vi "OpenCVCam_Stop.vi"(8 "ErrorIn":errorcluster, 10 "CmdData":variant, 11 "OpenCVCamIn":refnum<class>) -> (0 "ErrorOut":errorcluster, 2 "ReplyData":variant, 3 "OpenCVCamOut":refnum<class>, 4 "Exit":bool)   [LabVIEW 2021, in "OpenCVCam.lvclass"]
uses:
  OpenCVCam.lvclass
  OpenCVCam.lvclass/OpenCVCam.ctl
  State.ctl
  C:/Localdata/Projects/TriekselSoft/TriekselsoftApplicationFramework/Source/.Externals/Library_YAF/YAFTAF/YAFTAF.lvclass
  C:/Localdata/Projects/TriekselSoft/TriekselsoftApplicationFramework/Source/.Externals/Library_YAF/YActor/YActor.lvclass
  C:/Localdata/Projects/TriekselSoft/TriekselsoftApplicationFramework/Source/.Externals/Interface_UserInterface_IFrontPanel/IFrontPanel/IFrontPanel.lvclass
  C:/Localdata/Projects/TriekselSoft/TriekselsoftApplicationFramework/Source/IInterface/IInterface.lvclass
  C:/Localdata/Projects/TriekselSoft/TriekselsoftApplicationFramework/Source/.Externals/Interface_Object_ICreateDestroy/ICreateDestroy/ICreateDestroy.lvclass
  C:/Localdata/Projects/TriekselSoft/TriekselsoftApplicationFramework/Source/.Externals/Interface_Object_IPersistentData/IPersistentData/IPersistentData.lvclass
  C:/Localdata/Projects/TriekselSoft/TriekselsoftApplicationFramework/Source/.Externals/Interface_TAF_ITAFObject/ITAFObject/ITAFObject.lvclass
  C:/Localdata/Projects/TriekselSoft/TriekselsoftApplicationFramework/Source/YAFTAFObjects/OpenCVCam/OpenCVCam.lvclass
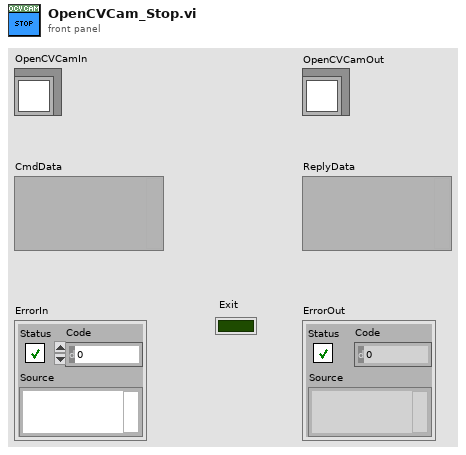
[diagram p1: front panel]
types:
  T1 = typedef "OpenCVCam.lvclass/State.ctl" = enum16{"Idle", "Initialized", "Acquiring"}
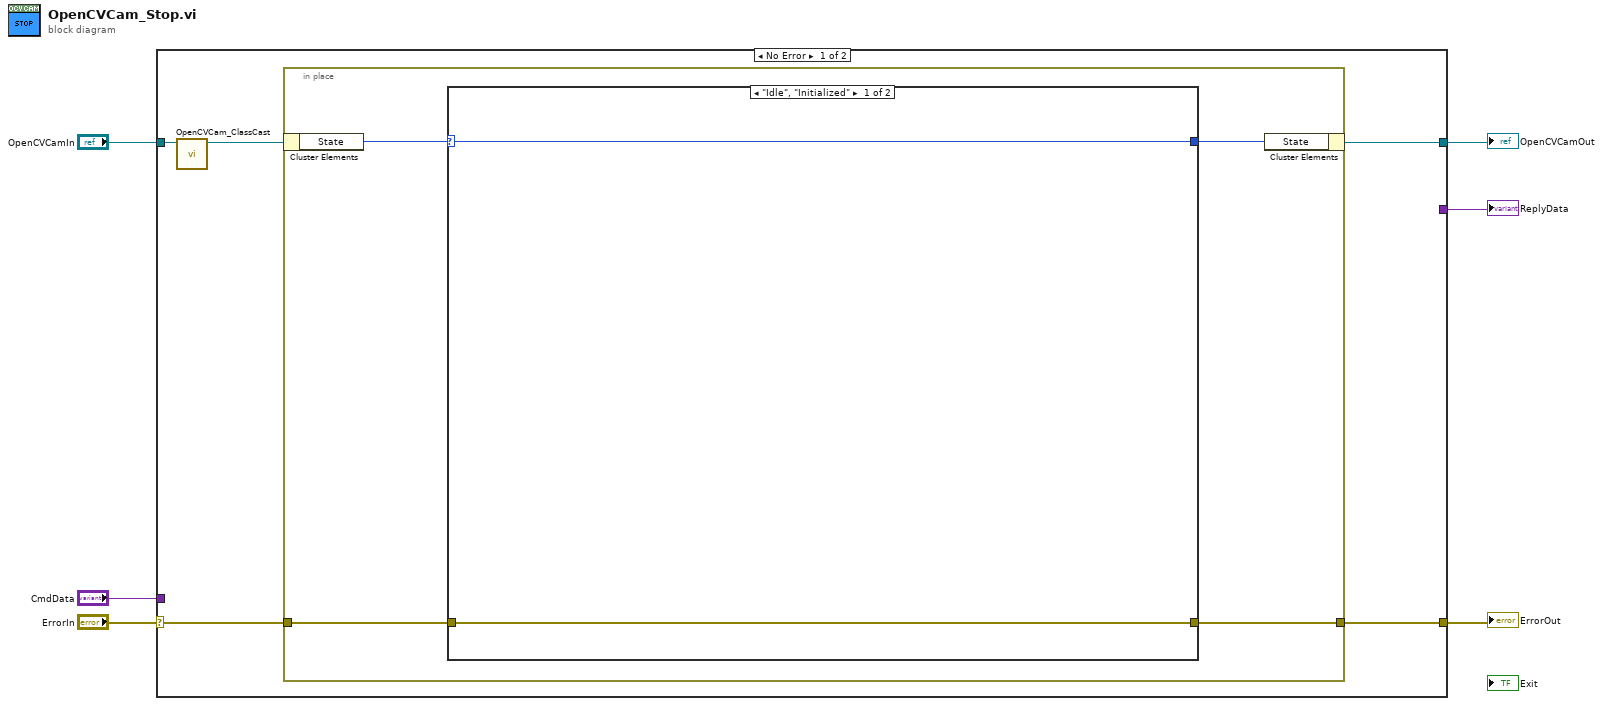
[diagram p0: block diagram]
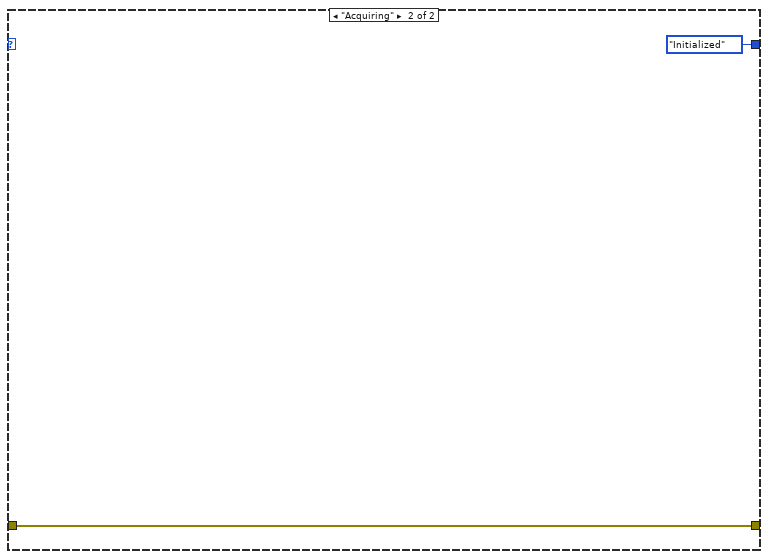
[diagram p2: hidden frame]
diagram:
  n1 = case shown="No Error" "ErrorIn" {
    selector: "ErrorIn" -> [w11 w22]
    tunnel: [w10 w22] -> w5
    tunnel: [_ w21] -> w3
    tunnel: "CmdData" -> [_ w21]
    tunnel: "OpenCVCamIn" -> [w9 w20]
    tunnel: [w7 w20] -> w1
    frame No Error {
      n2 = call "OpenCVCam_ClassCast.vi"("OpenCVCamIn"=w9) -> ("OpenCVCamOut"=w8:refnum<class "OpenCVCam.lvclass">)  [unwired: 10 in]
      n3 = in-place {
        in-place-border: w11 -> [w15]
        in-place-border: [w14] -> w10
        n4 = in-place-cluster #1(w8) -> ("State"=w13:T1)
        n5 = case shown="\"Idle\", \"Initialized\"" w13 {
          selector: w13 -> [w16 _]
          tunnel: [w17 w19] -> w14
          tunnel: w15 -> [w17 w19]
          tunnel: [w16 State."Initialized" ("State")] -> w12
          frame "Idle", "Initialized" {
          }
          frame "Acquiring" {
          }
        }
        n6 = in-place-cluster #1("State"=w12) -> (w7:refnum<class "OpenCVCam.lvclass">)
      }
    }
    frame Error {
    }
  }
  "ErrorOut" <- w5
  "OpenCVCamOut" <- w1
  "ReplyData" <- w3
